vi "find.vi"() -> ()   [LabVIEW 2020]
panel:
  out "find list":string[](array[string])
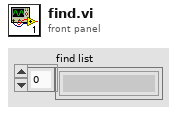
[diagram p1: front panel]
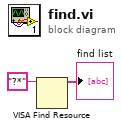
[diagram p0: block diagram]
diagram:
  n1 = VISA Find Resource(11:"?*" ("expression (\"?*\")")) -> (3:→"find list":string[])  [unwired: 2 in, 2 out]
